vi "ImageGrabEvent.vi"(4 "Callback Event":refnum<user-event>, 5 "Callback Param":cluster{"sender":refnum<k24>, "e":refnum<k24>}, 6 ".Control ref":refnum<k24>, 7 "Event Common Data":T1) -> ()   [LabVIEW 2013, in "GxLVlib.lvlib"]
uses:
  GxLVlib.lvlib
  F:/GxILibrary/Labview/trunk/private/dev/src/C#/x86/GxLVLib/dll/GxIAPINET.dll
  private/dev/src/C#/x86/GxLVLib/dll/GxIAPINET.dll
panel:
  out "error out":errorcluster
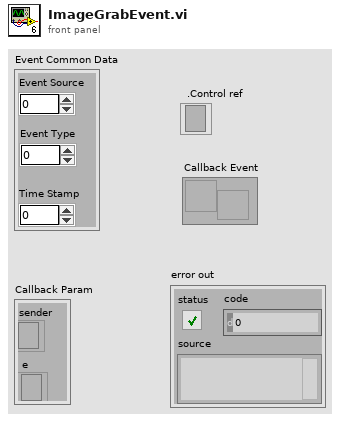
[diagram p1: front panel]
types:
  T1 = cluster{"Event Source":i32, "Event Type":u32, "Time Stamp":u32}
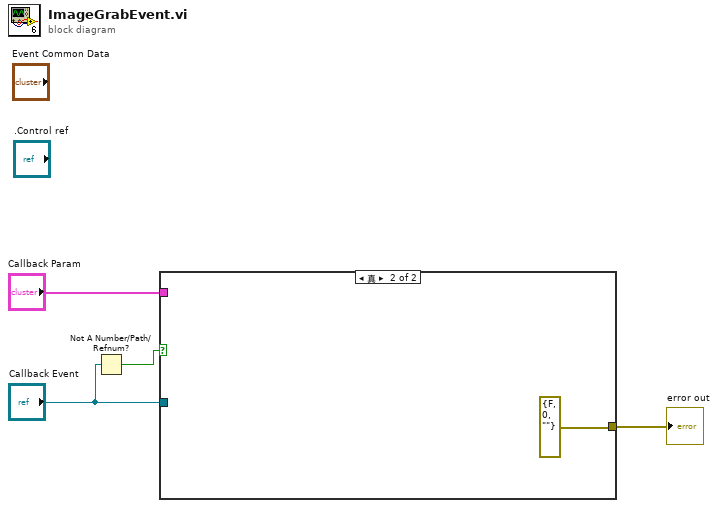
[diagram p0: block diagram]
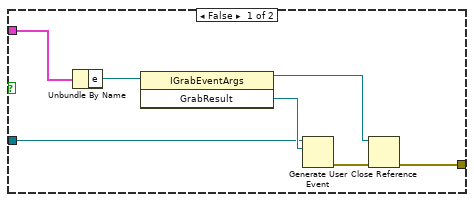
[diagram p2: hidden frame]
diagram:
  n1 = Not A Number/Path/Refnum?(number/path/refnum="Callback Event") -> (NaN/Path/Refnum?=w4:bool)
  n2 = case shown="真" w4 {
    tunnel: "Callback Event" -> [w8 _]
    tunnel: "Callback Param" -> [w10 _]
    tunnel: [w5 errorcluster {"status"=FALSE, "code"=0, "source"=""} ("错误常量")] -> w1
    frame False {
      n3 = Unbundle By Name(w10) -> ("e"=w11:refnum<k24>)
      n4 = invoke class="IGrabEventArgs" method="GrabResult"(reference=w11) -> (reference out=w6:refnum<k24>, "GrabResult"=w9:refnum<k24>)  [unwired: 2 in, 1 out]
      n5 = Generate User Event(user event=w8, event data cluster=w9) -> (error out=w7:errorcluster)  [unwired: 2 in, 1 out]
      n6 = Close Reference(reference=w6, error in (no error)=w7) -> (error out=w5:errorcluster)
    }
    frame True {
    }
  }
  "error out" <- w1
